vi "handle_CAN_error.vi"(11 "error in (no error)":errorcluster) -> (1 "stop":bool, 3 "error out":errorcluster)   [LabVIEW 2020]
uses:
  <vilib>/ErrorRing/Error Ring.xnode
panel:
  in  "retry delay (ms)":u32=300
  in  "# of tries":i32=5
  # "I think in my testing,\nthe 2nd attempt always worked\nso 3 is likely enough here.\nThat being said, better safe than sorry."
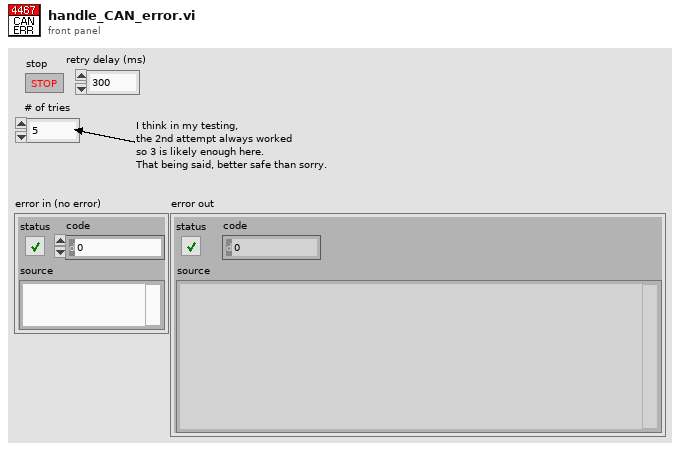
[diagram p1: front panel]
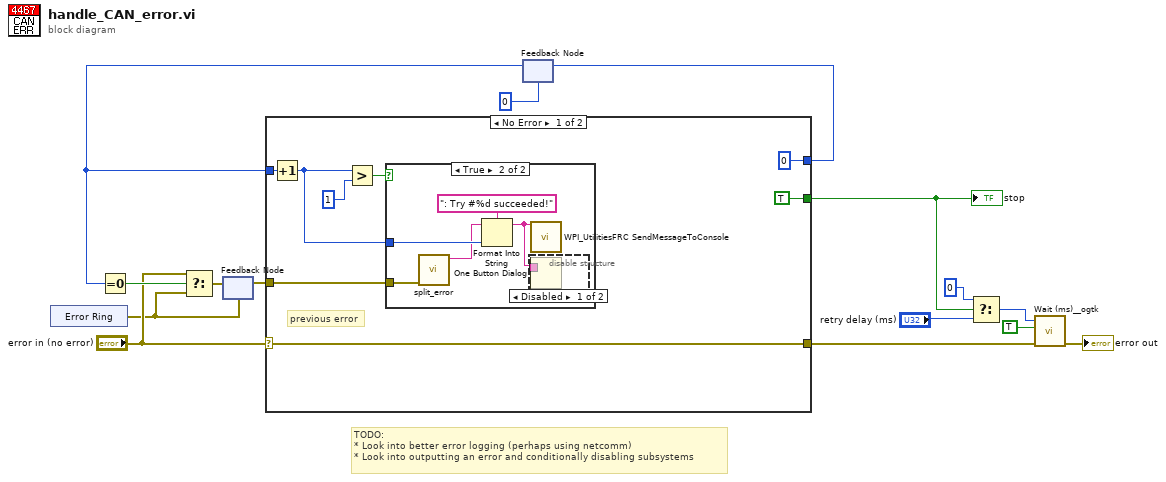
[diagram p0: block diagram]
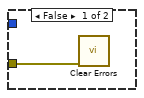
[diagram p2: hidden frame]
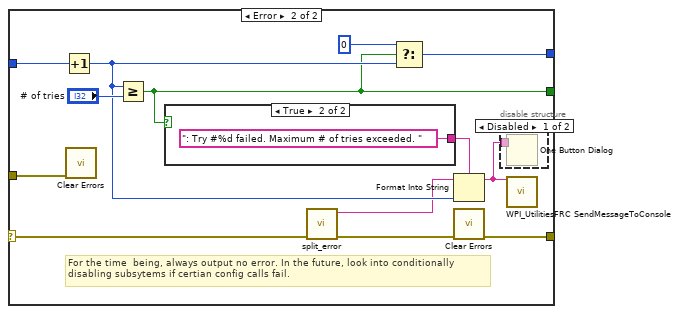
[diagram p4: hidden frame]
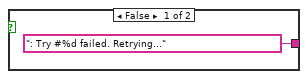
[diagram p6: hidden frame]
diagram:
  # "TODO:\n* Look into better error logging (perhaps using netcomm)\n* Look into outputting an error and conditionally disabling subsystems"
  n1 = xnode "Error Ring"() -> ("error out"=w3:errorcluster)
  n2 = feedback #1(w3) -> (w1:errorcluster)
  n3 = feedback #2(0) -> (w6:i32)
  n4 = Equal To 0?(x=w6) -> (x = 0?=w5:bool)
  n5 = Select(t="error in (no error)", s=w5, f=w3) -> (s? t:f=w2:errorcluster)
  n6 = feedback-in #1(w2) -> ()
  n7 = case shown="No Error" "error in (no error)" {
    selector: "error in (no error)" -> [w21 w36]
    tunnel: w6 -> [w20 w43]
    tunnel: [0 w40] -> w14
    tunnel: [TRUE ("stop") w33] -> w12
    tunnel: [w21 w31] -> w10
    tunnel: w1 -> [w17 w39]
    frame No Error {
      # "previous error"
      n8 = Increment(x=w20) -> (x+1=w18:i32)
      n9 = Greater?(x=w18, y=1) -> (0:w16:bool)
      n10 = case shown="True" w16 {
        tunnel: w18 -> [_ w29]
        tunnel: w17 -> [w24 w27]
        frame False {
          n11 = call <vilib>:"Clear Errors.vi"("error in (no error)"=w24) -> ()  [unwired: 5 in, 2 out]
        }
        frame True {
          n12 = call "split_error.vi"("error in"=w27) -> ("Details"=w26:string)  [unwired: 7 in, 3 out]
          n13 = Format Into String(format string=": Try #%d succeeded!" ("message"), initial string=w26, w29) -> (resulting string=w25:string)  [unwired: 1 in, 1 out]
          n14 = disable-structure shown="Disabled" {
            disable-tunnel: w25 -> [w30 _]
            frame Disabled {
              n15 = One Button Dialog(message=w30) -> ()  [unwired: 1 in, 1 out]
            }
            frame Enabled {
            }
          }
          n16 = call <vilib>:"WPI_UtilitiesFRC SendMessageToConsole.vi"("Message"=w25) -> ()  [unwired: 14 in, 1 out]
        }
      }
    }
    frame Error {
      # "For the time  being, always output no error. In the future, look into conditionally\ndisabling subsytems if certian config calls fail."
      n17 = Increment(x=w43) -> (x+1=w38:i32)
      n18 = call <vilib>:"Clear Errors.vi"("error in (no error)"=w39) -> ()  [unwired: 5 in, 2 out]
      n19 = Greater Or Equal?(x=w38, y="# of tries") -> (x >= y?=w33:bool)
      n20 = case shown="True" w33 {
        tunnel: [": Try #%d failed. Retrying..." ("message") ": Try #%d failed. Maximum # of tries exceeded. " ("message")] -> w37
        frame False {
        }
        frame True {
        }
      }
      n21 = call "split_error.vi"("error in"=w36) -> ("error out"=w32:errorcluster, "Details"=w35:string)  [unwired: 7 in, 2 out]
      n22 = Select(t=0, s=w33, f=w38) -> (s? t:f=w40:i32)
      n23 = Format Into String(format string=w37, initial string=w35, w38) -> (resulting string=w34:string)  [unwired: 1 in, 1 out]
      n24 = call <vilib>:"Clear Errors.vi"("error in (no error)"=w32) -> ("error out"=w31:errorcluster)  [unwired: 5 in, 1 out]
      n25 = disable-structure shown="Disabled" {
        disable-tunnel: w34 -> [w44 _]
        frame Disabled {
          n26 = One Button Dialog(message=w44) -> ()  [unwired: 1 in, 1 out]
        }
        frame Enabled {
        }
      }
      n27 = call <vilib>:"WPI_UtilitiesFRC SendMessageToConsole.vi"("Message"=w34) -> ()  [unwired: 14 in, 1 out]
    }
  }
  "stop" <- w12
  n28 = feedback-in #2(w14) -> ()
  n29 = Select(t=u32 0, s=w12, f="retry delay (ms)") -> (s? t:f=w7:u32)
  n30 = call "Wait (ms)__ogtk.vi"("error in (no error)"=w10, "Wait on Error (FALSE)"=TRUE, "milliseconds to wait"=w7) -> ("error out"=→"error out":errorcluster)  [unwired: 7 in, 1 out]
